vi "rethinkdb_tcp_read_null.vi"(6 "timeout ms (10000)":i32=10000, 8 "error in (no error)":errorcluster, 11 "rethinkdb in":refnum<k5>) -> (0 "error out":errorcluster, 2 "data out":string, 3 "rethinkdb out":refnum<k5>)   [LabVIEW 2017]
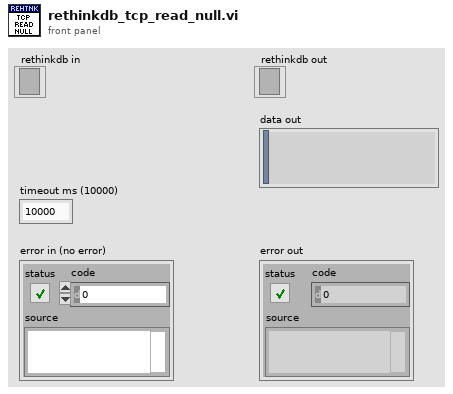
[diagram p1: front panel]
types:
  T1 = enum16{"Standard", "Buffered", "CRLF", "Immediate"}
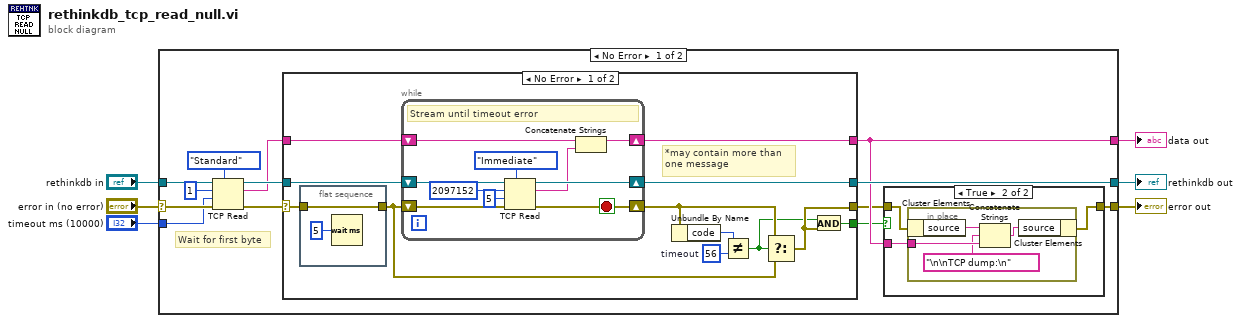
[diagram p0: block diagram]
diagram:
  n1 = case shown="No Error" "error in (no error)" {
    selector: "error in (no error)" -> [w18 w56]
    tunnel: "rethinkdb in" -> [w19 w55]
    tunnel: "timeout ms (10000)" -> [w17 _]
    tunnel: [w9 w56] -> w3
    tunnel: [w13 w55] -> w2
    tunnel: [w10 _] -> w1
    frame No Error {
      # "Wait for first byte"
      n2 = TCP Read(connection ID=w19, bytes to read=1, error in (no error)=w18, 7:T1."Standard" ("mode (standard)"), 9:w17) -> (connection ID out=w12:refnum<k5>, data out=w11:string, error out=w14:errorcluster)
      n3 = case shown="No Error" w14 {
        selector: w14 -> [w31 w46]
        tunnel: [w22 w46] -> w8
        tunnel: [w29 w45] -> w13
        tunnel: w12 -> [w30 w45]
        tunnel: w11 -> [w28 w44]
        tunnel: [w27 w44] -> w10
        tunnel: [w20 _] -> w7
        frame No Error {
          w25 = 56  # timeout
          # "*may contain more than\none message"
          n4 = flat-sequence {
            tunnel: [w42] -> w23
            tunnel: w31 -> [w42]
            frame #0 {
              n5 = Wait (ms)(milliseconds to wait=u32 5) -> ()  [unwired: 1 out]
            }
          }
          n6 = while {
            shift-right: [w33] -> w24
            shift-left: w23 -> [w41]
            shift-right: [w39] -> w29
            shift-left: w30 -> [w40]
            shift-right: [w32] -> w27
            shift-left: w28 -> [w35]
            stop <- w33 stop-if-true
            # "Stream until timeout error"
            n7 = TCP Read(connection ID=w40, bytes to read=2097152, error in (no error)=w41, 7:T1."Immediate" ("mode (standard)"), 9:5 ("timeout ms (25000)")) -> (connection ID out=w39:refnum<k5>, data out=w34:string, error out=w33:errorcluster)
            n8 = Concatenate Strings(w35, w34) -> (w32:string)
          }
          n9 = Unbundle By Name(w24) -> ("code"=w26:i32)
          n10 = Not Equal?(x=w26, y=w25) -> (x != y?=w21:bool)
          n11 = Select(t=w24, s=w21, f=w23) -> (s? t:f=w22:errorcluster)
          n12 = And(x=w21, y=w22) -> (x .and. y?=w20:bool)
        }
        frame Error {
        }
      }
      n13 = case shown="True" w7 {
        tunnel: w10 -> [_ w50]
        tunnel: [w47 w49] -> w9
        tunnel: w8 -> [w47 w48]
        frame False {
        }
        frame True {
          n14 = in-place {
            in-place-border: w50 -> [w52]
            n15 = in-place-cluster #1(w48) -> ("source"=w54:string)
            n16 = Concatenate Strings(w54, "\n\nTCP dump:\n" ("format string"), w52) -> (w53:string)
            n17 = in-place-cluster #1("source"=w53) -> (w49:errorcluster)
          }
        }
      }
    }
    frame Error {
    }
  }
  "error out" <- w3
  "rethinkdb out" <- w2
  "data out" <- w1
